vi "Apply Property.vi"(0 "TTLControl in":refnum<class "TCPController.lvclass">, 5 "TTL name":string, 7 "param":string, 9 "value":dbl, 11 "error in (no error)":errorcluster) -> (4 "TTLControl out":refnum<class "TCPController.lvclass">, 8 "Disabled":bool, 15 "error out":errorcluster)   [LabVIEW 2020, in "TCPController.lvclass"]
uses:
  TCPController.lvclass
  D:/Development/epl-tosca/LV Source/TTL VIs/Control Classes/Base Class/TTLController.lvclass
  Base Class/TTLController.lvclass/TTLController.ctl
  TCPController.lvclass/TCPController.ctl
  Write Value 2.vi
  Write Value.vi
  Base Class/Read Name.vi
  Base Class/TTLController.lvclass
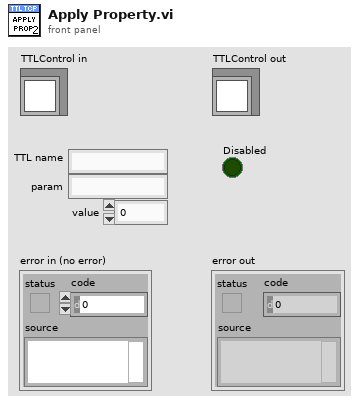
[diagram p1: front panel]
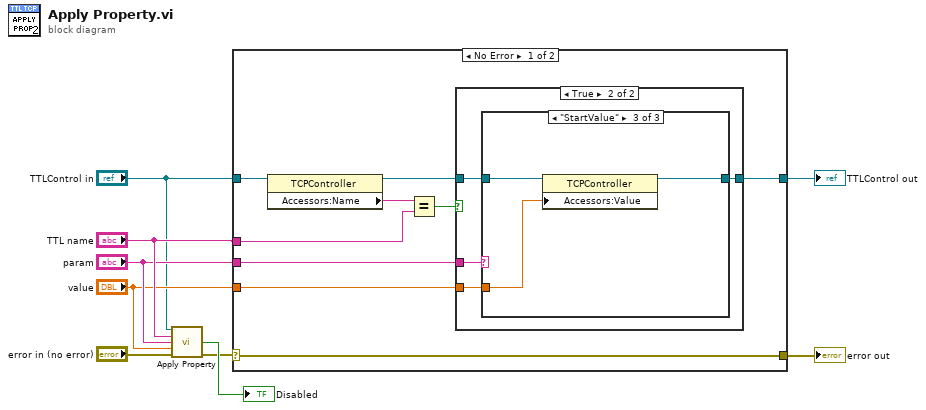
[diagram p0: block diagram]
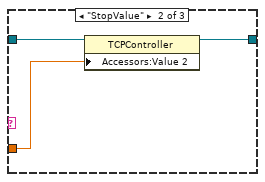
[diagram p4: hidden frame]
diagram:
  n1 = call-parent "Apply Property.vi"("TTLControl in"="TTLControl in", "TTL name"="TTL name", "param"="param", "value"="value", "error in (no error)"="error in (no error)") -> ("Disabled"=→"Disabled":bool, "error out"=w7:errorcluster)  [unwired: 8 in, 1 out]
  n2 = case shown="No Error" w7 {
    selector: w7 -> [w18 w32]
    tunnel: [w18 w32] -> w1
    tunnel: [w13 w31] -> w2
    tunnel: "TTLControl in" -> [w12 w31]
    tunnel: "TTL name" -> [w16 _]
    tunnel: "param" -> [w15 _]
    tunnel: "value" -> [w14 _]
    frame No Error {
      n3 = property class="TCPController"(reference=w12) -> (reference out=w11:refnum<class "TCPController.lvclass">, "Accessors:Name"=w10:string)  [unwired: 1 in, 1 out]
      n4 = Equal?(x=w10, y=w16) -> (x = y?=w17:bool)
      n5 = case shown="True" w17 {
        tunnel: w11 -> [w19 w23]
        tunnel: [w19 w22] -> w13
        tunnel: w14 -> [_ w21]
        tunnel: w15 -> [_ w20]
        frame False {
        }
        frame True {
          n6 = case shown="\"StartValue\"" w20 {
            tunnel: w23 -> [w24 w27 w30]
            tunnel: [w24 w26 w29] -> w22
            tunnel: w21 -> [_ w25 w28]
            frame "", Default {
            }
            frame "StopValue" {
              n7 = property class="TCPController"(reference=w27, "Accessors:Value 2"=w25) -> (reference out=w26:refnum<class "TCPController.lvclass">)  [unwired: 1 in, 1 out]
            }
            frame "StartValue" {
              n8 = property class="TCPController"(reference=w30, "Accessors:Value"=w28) -> (reference out=w29:refnum<class "TCPController.lvclass">)  [unwired: 1 in, 1 out]
            }
          }
        }
      }
    }
    frame Error {
    }
  }
  "error out" <- w1
  "TTLControl out" <- w2
